vi "TPNT_CheckLimitConsistecy.vi"(8 "error in (no error)":errorcluster, 9 "lower":dbl format="%.2f", 10 "nominal":dbl format="%.2f", 11 "upper":dbl format="%.2f") -> (0 "error out":errorcluster, 2 "OK?":bool, 3 "message":string="ERROR Lower limit is greater than upper limit")   [LabVIEW 2016]
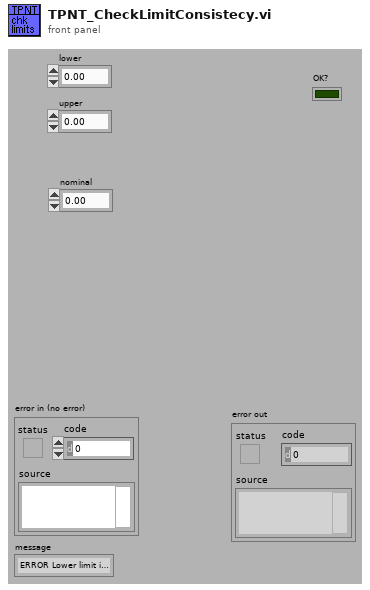
[diagram p1: front panel]
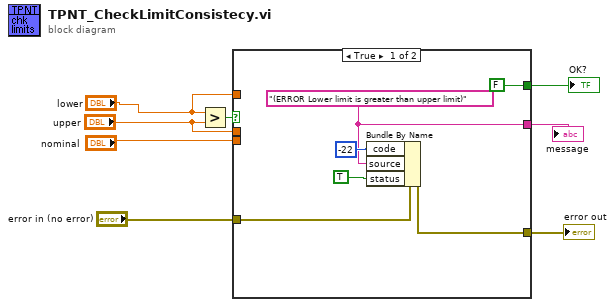
[diagram p0: block diagram]
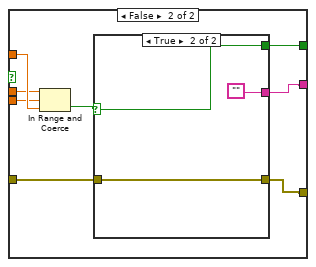
[diagram p2: hidden frame]
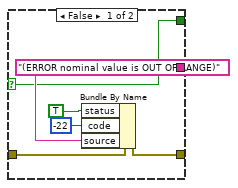
[diagram p3: hidden frame]
diagram:
  n1 = Greater?(x="lower", y="upper") -> (0:w8:bool)
  n2 = case shown="True" w8 {
    tunnel: "error in (no error)" -> [w14 w18]
    tunnel: [w13 w17] -> w6
    tunnel: "lower" -> [_ w21]
    tunnel: "upper" -> [_ w20]
    tunnel: "nominal" -> [_ w19]
    tunnel: [w10 w16] -> w2
    tunnel: [FALSE w15] -> w1
    frame True {
      w10 = "(ERROR Lower limit is greater than upper limit)"
      n3 = Bundle By Name(cluster=w14, "code"=-22, "source"=w10, "status"=TRUE) -> (w13:errorcluster)
    }
    frame False {
      n4 = In Range and Coerce(upper limit=w20, x=w19, lower limit=w21) -> (In Range?=w22:bool)  [unwired: 1 out]
      n5 = case shown="True" w22 {
        selector: w22 -> [w23 w29]
        tunnel: w18 -> [w28 w31]
        tunnel: [w27 w31] -> w17
        tunnel: [w24 ""] -> w16
        tunnel: [w23 w29] -> w15
        frame False {
          w24 = "(ERROR nominal value is OUT OF RANGE)"
          n6 = Bundle By Name(cluster=w28, "status"=TRUE, "code"=-22, "source"=w24) -> (w27:errorcluster)
        }
        frame True {
        }
      }
    }
  }
  "error out" <- w6
  "OK?" <- w1
  "message" <- w2
